vi "format_to_uncertainty.vi"(7 "Separate thousands":bool, 8 "unit":string, 9 "Add SI prefix (true)":bool=TRUE, 10 "uncertainty":dbl format="%#_6p", 11 "value":dbl format="%#_6p") -> (0 "SI prefix and unit string":string, 1 "uncertainty string":string, 2 "value string":string, 3 "string out":string)   [LabVIEW 2020, in "varilib.lvlib"]
doc: "This VI combines value, uncertainty and unit into combined string formated to two significant digits. The VI also supports scaling by SI prefixes. Output format example: (1.0059 ± 0.0022) mV. SI prefix scaling can be disabled which may be usefull for unitless quantities."
uses:
  varilib.lvlib
  <vilib>/regexp/Match Regular Expression.xnode
panel:
  out "number format":string
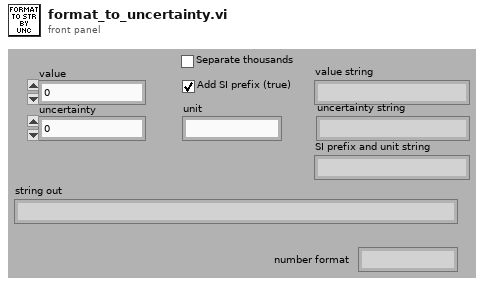
[diagram p1: front panel]
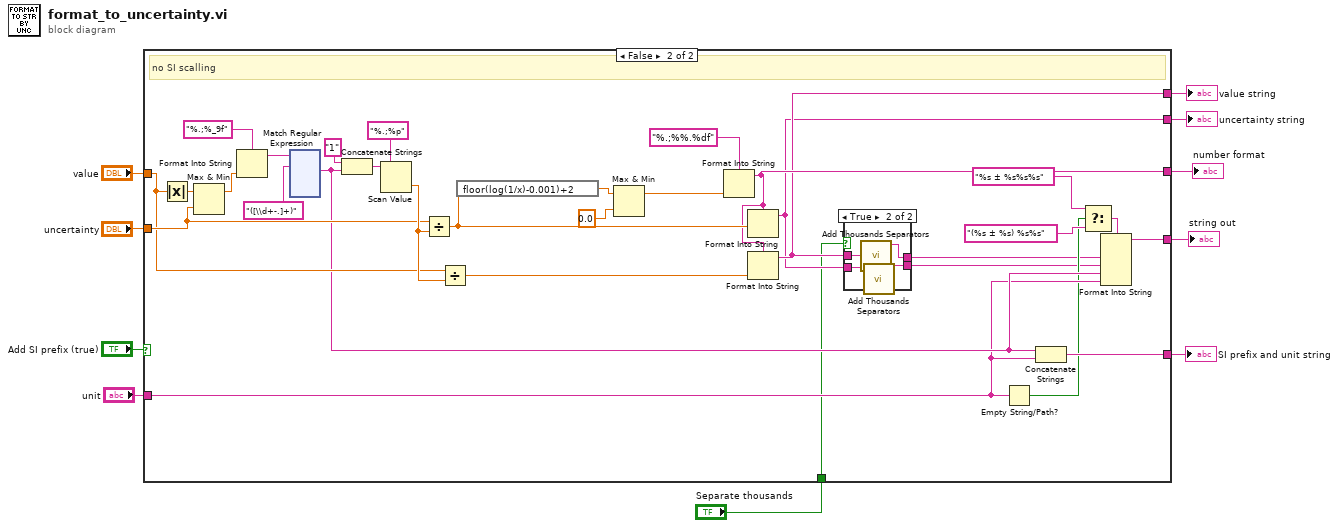
[diagram p0: block diagram]
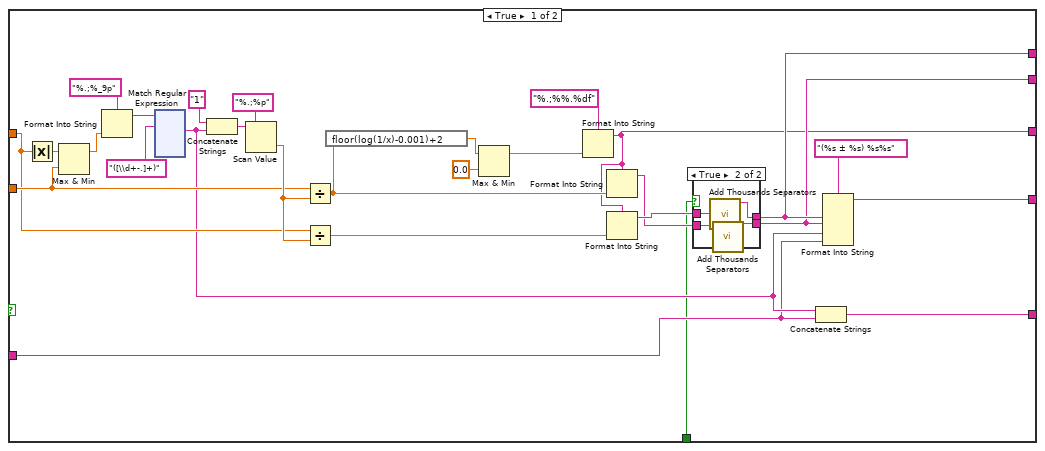
[diagram p2: hidden frame]
diagram:
  n1 = case shown="False" "Add SI prefix (true)" {
    tunnel: "value" -> [w24 w178]
    tunnel: "uncertainty" -> [w25 w179]
    tunnel: [w26 w180] -> w8
    tunnel: "unit" -> [w18 w169]
    tunnel: [w15 w164] -> w5
    tunnel: [w14 w163] -> w4
    tunnel: [w20 w173] -> w3
    tunnel: [w13 w167] -> w2
    tunnel: "Separate thousands" -> [w11 w161]
    frame True {
      n2 = Absolute Value(x=w24) -> (abs(x)=w21:dbl)
      n3 = Max & Min(x=w21, y=w25) -> (max(x,y)=w23:dbl)  [unwired: 1 out]
      n4 = Format Into String(format string="%.;%_9p", w23) -> (resulting string=w38:string)  [unwired: 2 in, 1 out]
      n5 = xnode "Match Regular Expression"("input string"=w38, "regular expression"="([\\d+-.]+)") -> ("after match"=w19:string)  [unwired: 4 in, 5 out]
      n6 = Concatenate Strings("1" ("string"), w19) -> (w35:string)
      n7 = Scan Value(string=w35, format string="%.;%p") -> (value=w31:dbl)  [unwired: 1 in, 1 out]
      n8 = Divide(x=w25, y=w31) -> (x/y=w29:dbl)
      n9 = Divide(x=w24, y=w31) -> (x/y=w30:dbl)
      n10 = expression code="floor(log(1/x)-0.001)+2"(w29) -> (w33:dbl)
      n11 = Max & Min(x=w33, y=0.0) -> (max(x,y)=w12:dbl)  [unwired: 1 out]
      n12 = Format Into String(format string="%.;%%.%df", w12) -> (resulting string=w13:string)  [unwired: 2 in, 1 out]
      n13 = Format Into String(format string=w13, w29) -> (resulting string=w16:string)  [unwired: 2 in, 1 out]
      n14 = Format Into String(format string=w13, w30) -> (resulting string=w17:string)  [unwired: 2 in, 1 out]
      n15 = case shown="True" w11 {
        tunnel: w17 -> [w39 w44]
        tunnel: [w39 w43] -> w15
        tunnel: w16 -> [w40 w42]
        tunnel: [w40 w41] -> w14
        frame False {
        }
        frame True {
          n16 = call "Add Thousands Separators.vi"("Number as string"=w44) -> ("Number as separated string"=w43:string)  [unwired: 10 in]
          n17 = call "Add Thousands Separators.vi"("Number as string"=w42) -> ("Number as separated string"=w41:string)  [unwired: 10 in]
        }
      }
      n18 = Concatenate Strings(w19, w18) -> (w20:string)
      n19 = Format Into String(format string="(%s ± %s) %s%s", w15, w14, w19, w18) -> (resulting string=w26:string)  [unwired: 2 in, 1 out]
    }
    frame False {
      # "no SI scalling"
      n20 = Absolute Value(x=w178) -> (abs(x)=w175:dbl)
      n21 = Max & Min(x=w175, y=w179) -> (max(x,y)=w177:dbl)  [unwired: 1 out]
      n22 = Format Into String(format string="%.;%_9f", w177) -> (resulting string=w191:string)  [unwired: 2 in, 1 out]
      n23 = xnode "Match Regular Expression"("input string"=w191, "regular expression"="([\\d+-.]+)") -> ("after match"=w174:string)  [unwired: 4 in, 5 out]
      n24 = Concatenate Strings("1" ("string"), w174) -> (w188:string)
      n25 = Scan Value(string=w188, format string="%.;%p") -> (value=w184:dbl)  [unwired: 1 in, 1 out]
      n26 = Divide(x=w179, y=w184) -> (x/y=w182:dbl)
      n27 = Divide(x=w178, y=w184) -> (x/y=w183:dbl)
      n28 = expression code="floor(log(1/x)-0.001)+2"(w182) -> (w186:dbl)
      n29 = Max & Min(x=w186, y=0.0) -> (max(x,y)=w166:dbl)  [unwired: 1 out]
      n30 = Format Into String(format string="%.;%%.%df", w166) -> (resulting string=w167:string)  [unwired: 2 in, 1 out]
      n31 = Format Into String(format string=w167, w182) -> (resulting string=w163:string)  [unwired: 2 in, 1 out]
      n32 = Format Into String(format string=w167, w183) -> (resulting string=w164:string)  [unwired: 2 in, 1 out]
      n33 = case shown="True" w161 {
        tunnel: w164 -> [w192 w197]
        tunnel: [w192 w196] -> w165
        tunnel: w163 -> [w193 w195]
        tunnel: [w193 w194] -> w162
        frame False {
        }
        frame True {
          n34 = call "Add Thousands Separators.vi"("Number as string"=w197) -> ("Number as separated string"=w196:string)  [unwired: 10 in]
          n35 = call "Add Thousands Separators.vi"("Number as string"=w195) -> ("Number as separated string"=w194:string)  [unwired: 10 in]
        }
      }
      n36 = Empty String/Path?(string/path=w169) -> (empty?=w168:bool)
      n37 = Concatenate Strings(w174, w169) -> (w173:string)
      n38 = Select(t="%s ± %s%s%s" ("format string"), s=w168, f="(%s ± %s) %s%s" ("format string")) -> (s? t:f=w172:string)
      n39 = Format Into String(format string=w172, w165, w162, w174, w169) -> (resulting string=w180:string)  [unwired: 2 in, 1 out]
    }
  }
  "string out" <- w8
  "value string" <- w5
  "uncertainty string" <- w4
  "SI prefix and unit string" <- w3
  "number format" <- w2
